vi "EXO1_DataRead&Plot.vi"() -> ()   [LabVIEW 2012]
uses:
  <vilib>/addons/database/Connection.llb/DB Tools Open Connec (Path).vi
  <vilib>/addons/database/NI_Database_API.lvlib
panel:
  out "element":string
  out "error out 2":errorcluster
  in  "Tree 2":string[](tree)=["170: Buffer Volume High Pressure Limit (torr)"]
  out "Plot":cluster{dbl[], dbl[]}(graph)
  in  "Start time":timestamp
  in  "End time":timestamp
  out "Data List":string[][](table)
  out "error out":errorcluster
  in  "Table chosen":string="EXO"
  in  "stop":bool
  # "EXO Data Read & Plots"
  # "Select Data Channel"
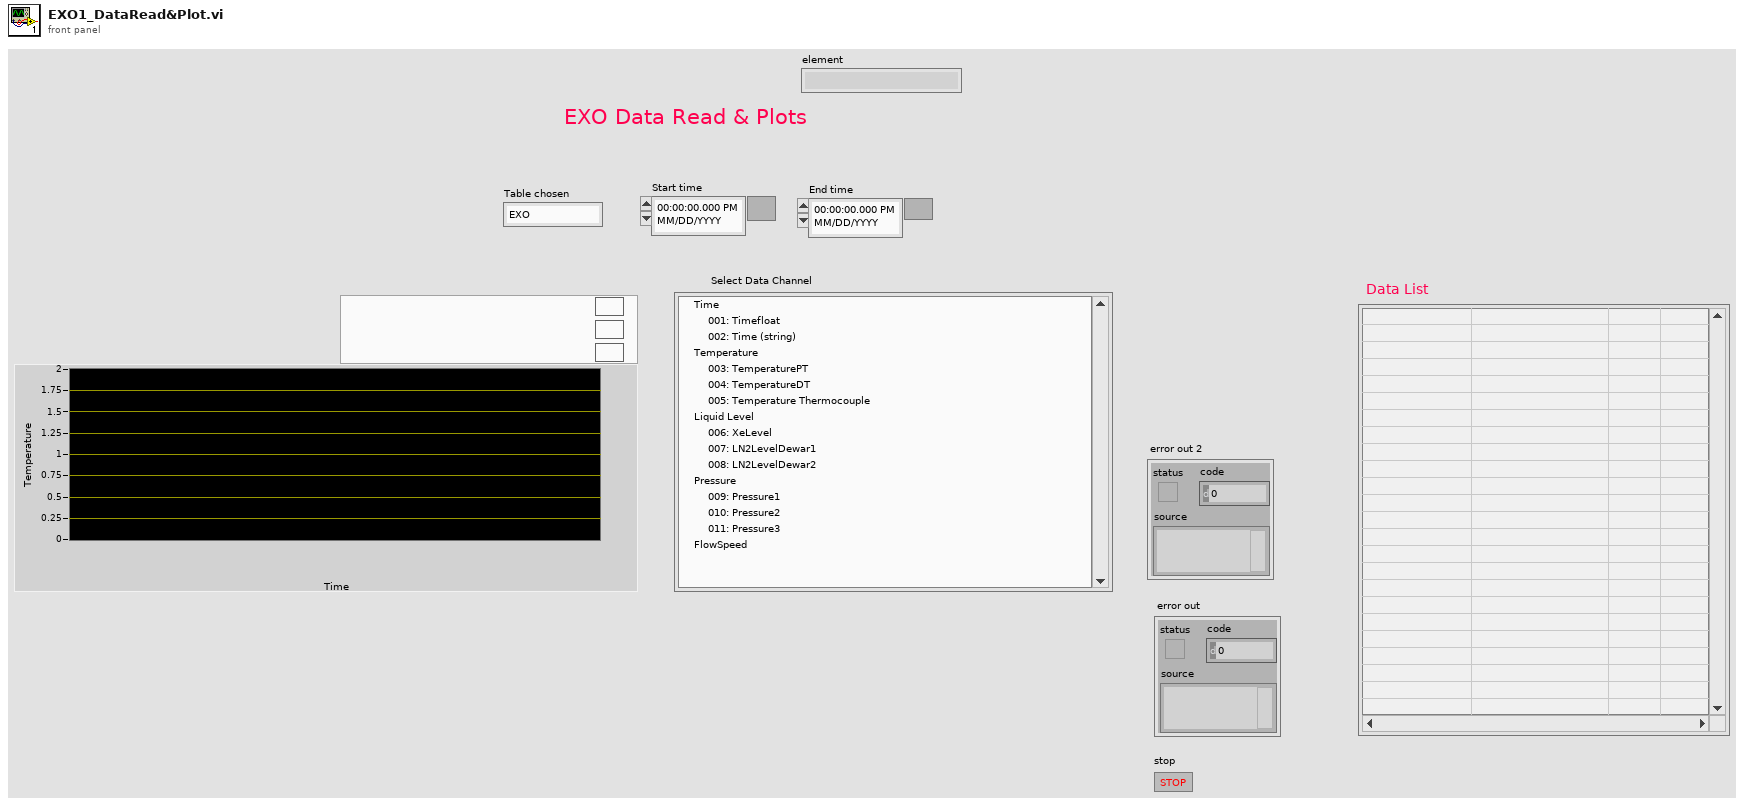
[diagram p1: front panel]
types:
  T1 = typedef "NI_Database_API.lvlib/Conn ObjectReference.ctl" = refnum<k1>
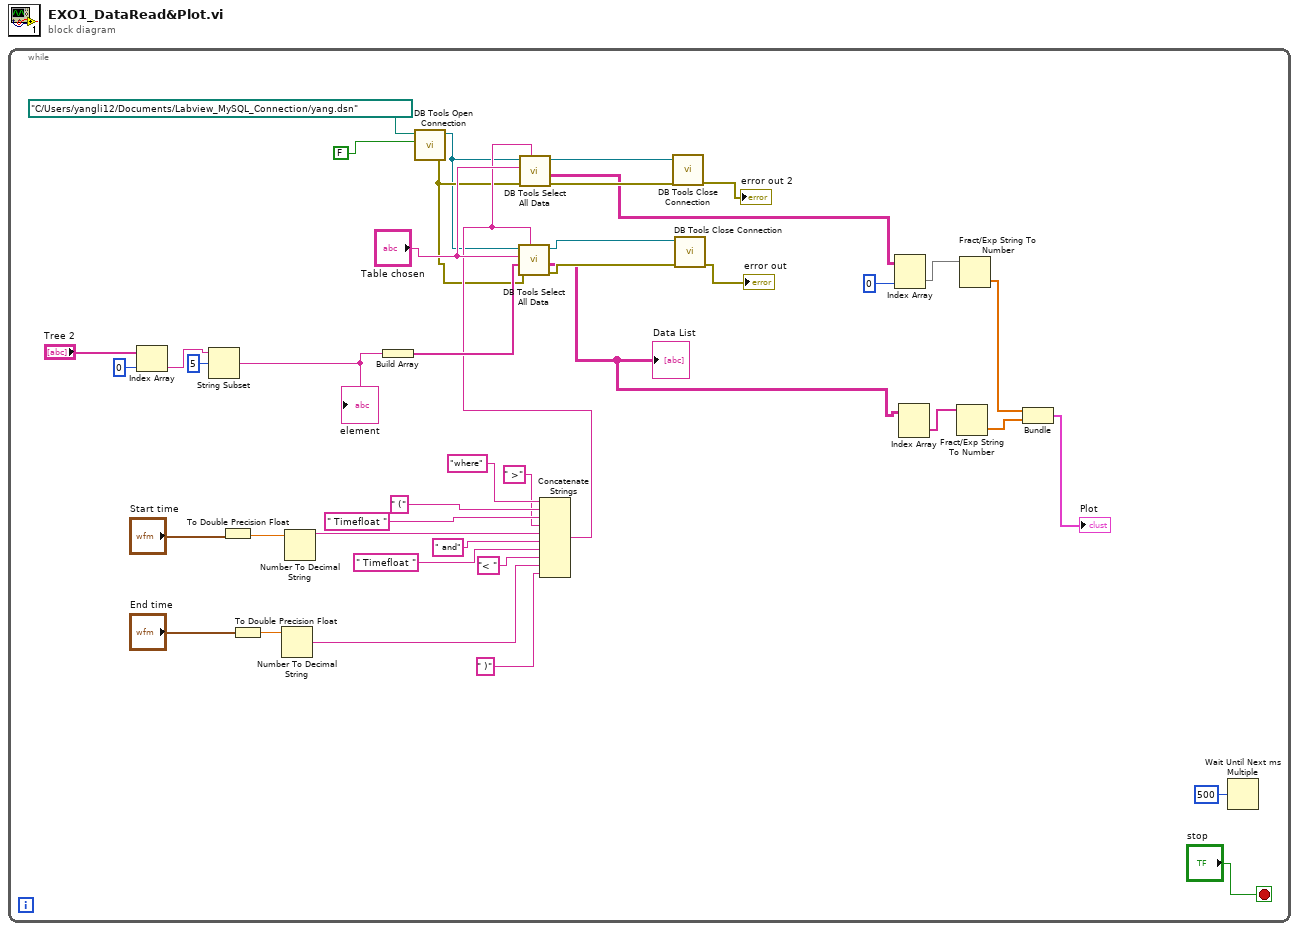
[diagram p0: block diagram]
diagram:
  n1 = while {
    stop <- "stop" stop-if-true
    n2 = Index Array(array="Tree 2", index=0) -> (element=w2:string)
    n3 = String Subset(string=w2, offset (0)=5) -> (substring=w1:string)  [unwired: 1 in]
    "element" <- w1
    n4 = To Double Precision Float(number="Start time") -> (double precision float=w29:dbl)
    n5 = To Double Precision Float(number="End time") -> (double precision float=w24:dbl)
    n6 = Number To Decimal String(number=w24) -> (decimal integer string=w23:string)  [unwired: 1 out]
    n7 = Number To Decimal String(number=w29) -> (decimal integer string=w28:string)  [unwired: 1 out]
    n8 = Build Array(w1) -> (w20:string[])
    n9 = call-poly <vilib>:"DB Tools Open Connection.vi"("prompt? (F)"=FALSE, "connection information"=path "C:/Users/yangli12/Documents/Labview_MySQL_Connection/yang.dsn") -> ("error out"=w13:errorcluster, "connection reference"=w5:T1)  [unwired: 6 in]
    n10 = Concatenate Strings("where", " (", " Timefloat " ("string"), " >" ("string"), w28, " and", " Timefloat ", "< " ("string"), w23, " )") -> (w14:string)
    n11 = call <vilib>:"DB Tools Select All Data.vi"("optional clause"=w14, "error in (no error)"=w13, "columns"=w20, "table"="Table chosen", "connection reference"=w5) -> ("error out"=w37:errorcluster, "data"=w7:string[][], "connection reference out"=w36:T1)  [unwired: 1 out]
    "Data List" <- w7
    n12 = call <vilib>:"DB Tools Select All Data.vi"("optional clause"=w14, "error in (no error)"=w13, "table"="Table chosen", "connection reference"=w5) -> ("error out"=w17:errorcluster, "data"=w12:string[][], "connection reference out"=w16:T1)  [unwired: 1 in, 1 out]
    n13 = call <vilib>:"DB Tools Close Connection.vi"("error in (no error)"=w17, "connection reference"=w16) -> ("error out"=→"error out 2":errorcluster)  [unwired: 5 in]
    n14 = call <vilib>:"DB Tools Close Connection.vi"("error in (no error)"=w37, "connection reference"=w36) -> ("error out"=→"error out":errorcluster)  [unwired: 5 in]
    n15 = Index Array(array=w12, index (col)=0 ("disabled index (col)")) -> (element=w10:string[])  [unwired: 1 in]
    n16 = Index Array(array=w7) -> (element=w6:string[])  [unwired: 2 in]
    n17 = Fract/Exp String To Number(string=w6) -> (number=w19:dbl[])  [unwired: 4 out]
    n18 = Fract/Exp String To Number(string=w10) -> (number=w9:dbl[])  [unwired: 4 out]
    n19 = Bundle "Bundle"(w9, w19) -> (→"Plot":cluster{dbl[], dbl[]})  [unwired: 1 in]
    n20 = Wait Until Next ms Multiple(millisecond multiple=u32 500) -> ()  [unwired: 1 out]
  }
